vi "3-lorentzian-heat-response -- V4.vi"(7 "action":T2, 10 "Map IN":map{T1, dbl}(c390), 11 "omega IN (rad/sec)":dbl=0.1 format="%#_10f") -> (1 "Romega":cdb=0.1+0.0i format="%#_10f", 2 "Map OUT":map{T1, dbl}(c390), 3 "omega OUT(rad/sec)":dbl=0.1 format="%#_10f")   [LabVIEW 2020]
uses:
  3-lorentzian-heat-response action.ctl
  3-lorentzian-parameters.ctl
  142dd4c5-f9ed-c64b-bc14-a88e3e2c450a.vi
  <vilib>/Analysis/polynomials.llb/Polynomial Roots (DBL).vi
  <vilib>/Comparison/Less/Less Functor/Less Functor.lvclass
  <vilib>/Analysis/NI_AALPro.lvlib
panel:
  out "m1":dbl=0.1 format="%#_10f"
  out "m2":dbl=0.1 format="%#_10f"
  out "m3":dbl=0.1 format="%#_10f"
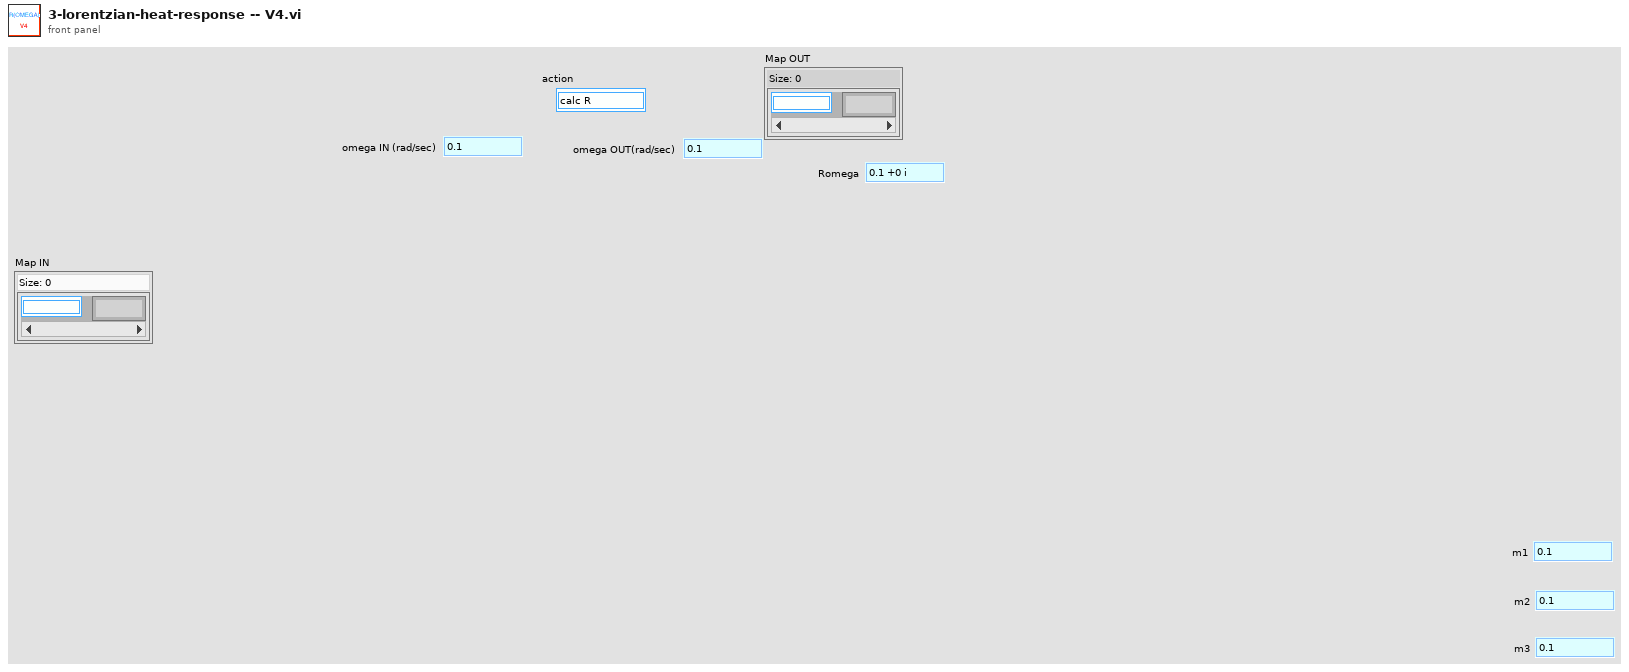
[diagram p1: front panel]
types:
  T1 = typedef "3-lorentzian-parameters.ctl" = enum16{"ζ", "τ1", "τS", "τN", "τC", "κ0", "m1", "m2", "m3", "T (K)", "B (T)", "θ (deg)", "side (S|R)", "set of (B|T)", "Re(offset)", "Im(offset)"}
  T2 = typedef "3-lorentzian-heat-response action.ctl" = enum16{"calc R", "create string", "calc m1m2m3", "dζ", "dT1", "dτS", "dτN", "dτC", "d-all", "dκ0", "T(K)", "m1", "m2", "m3", "parse string", "θ (deg)", "B (T)", "onlygrads", "newton", "create emty string"}
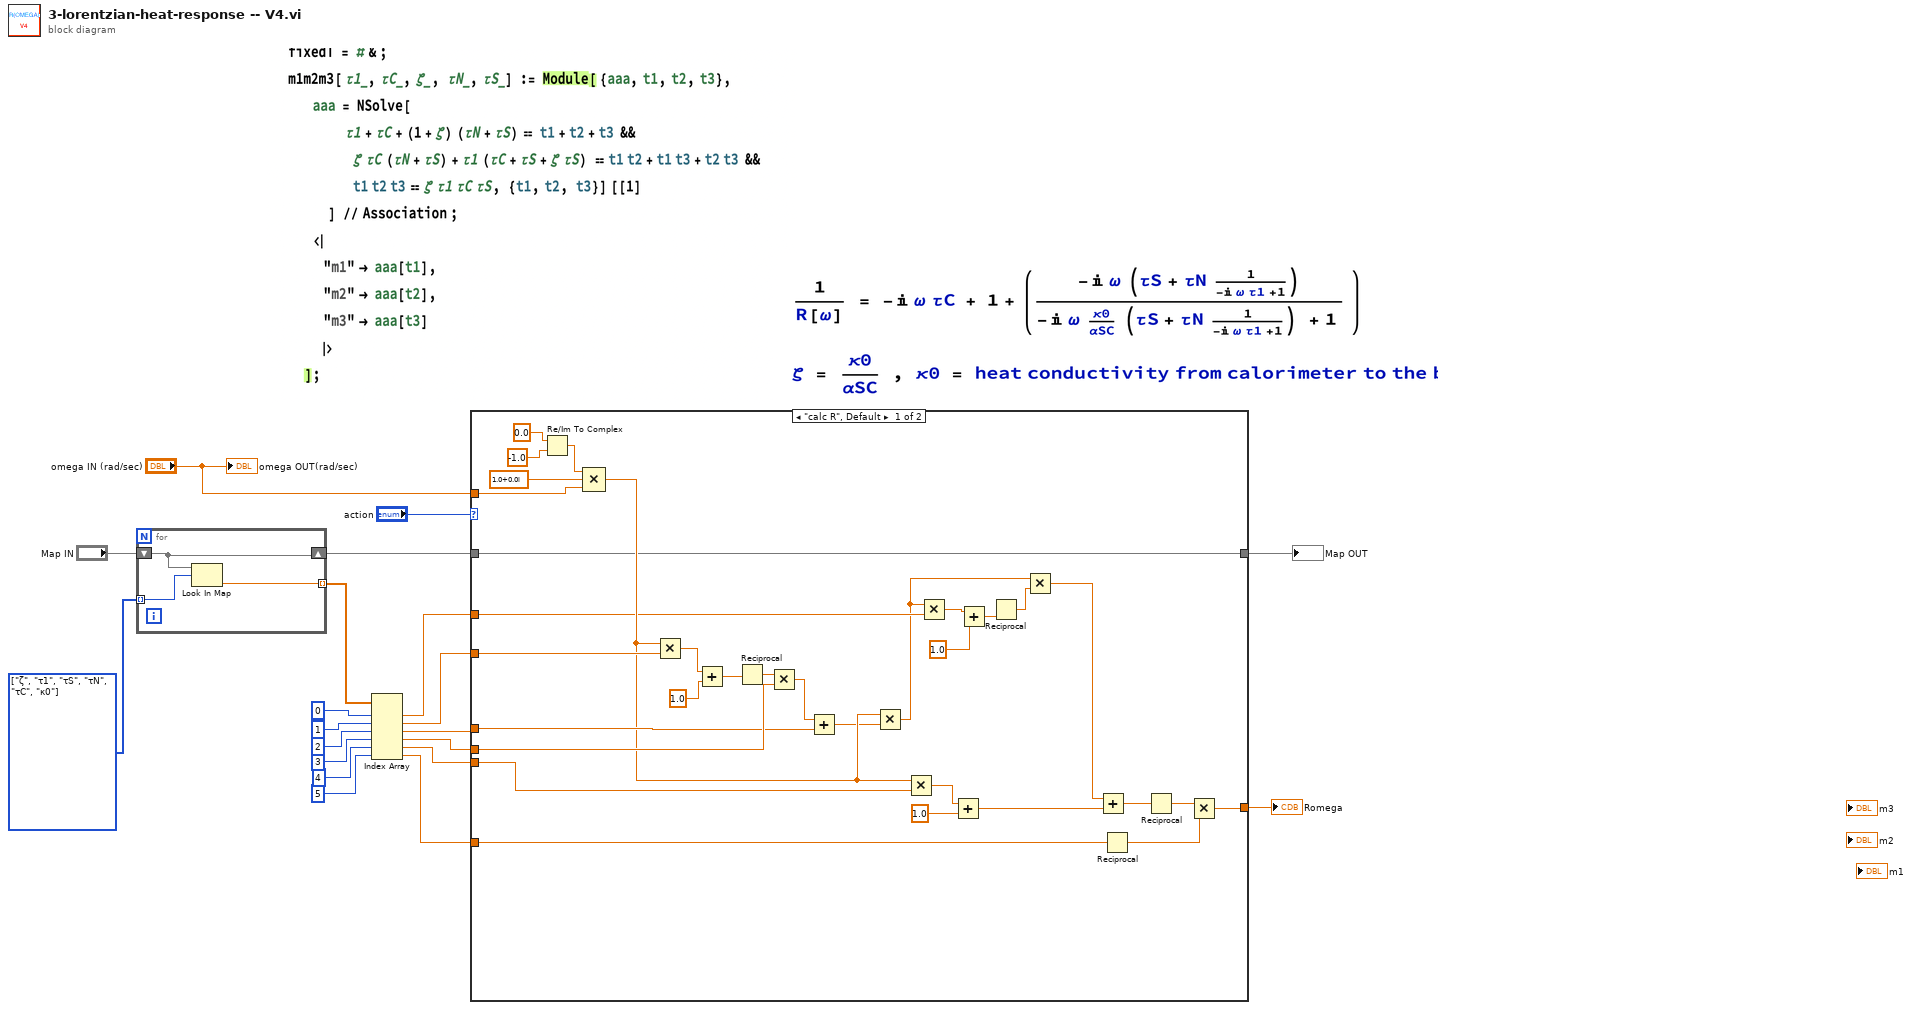
[diagram p0: block diagram]
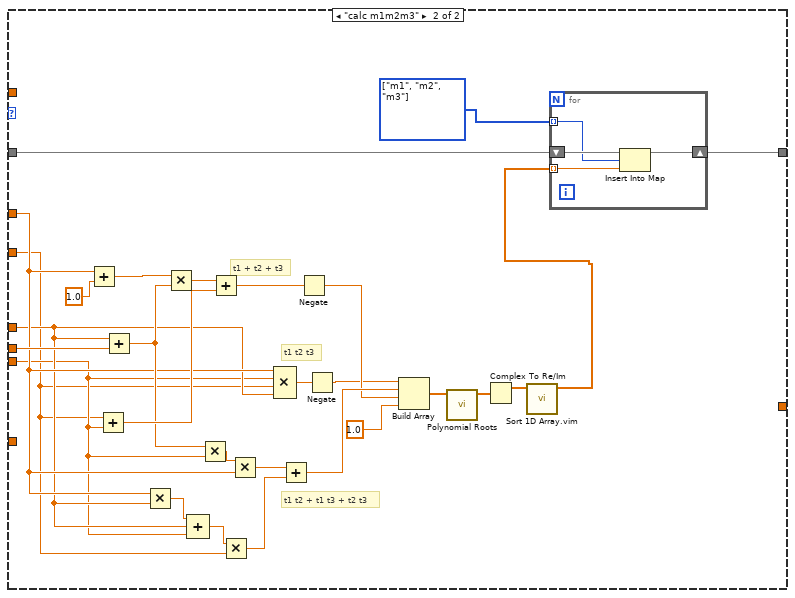
[diagram p2: hidden frame]
diagram:
  w5 = T1[] [enum."ζ", enum."τ1", enum."τS", enum."τN", enum."τC", enum."κ0"] items=["ζ", "τ1", "τS", "τN", "τC", "κ0", "m1", "m2", "m3", "T (K)", "B (T)", "θ (deg)", "side (S|R)", "set of (B|T)", "Re(offset)", "Im(offset)"]
  n1 = for {
    tunnel: w5 -> [w23] mode=indexing
    tunnel: [w22] -> w3 mode=indexing
    shift-right: [w21] -> w2
    shift-left: "Map IN" -> [w21]
    n2 = Look In Map(map=w21, key=w23) -> (value=w22:dbl)  [unwired: 1 in, 1 out]
  }
  n3 = Index Array(array=w3, index #1=0 ("index"), index #2=1 ("index"), index #3=2 ("index"), index #4=3 ("index"), index #5=4 ("index"), index #6=5 ("index")) -> (element #1=w12:dbl, element #2=w11:dbl, element #3=w10:dbl, element #4=w9:dbl, element #5=w8:dbl, element #6=w7:dbl)
  n4 = case shown="\"calc R\", Default" "action" {
    tunnel: w8 -> [w41 w69]
    tunnel: "omega IN (rad/sec)" -> [w44 _]
    tunnel: w11 -> [w43 w67]
    tunnel: w9 -> [w49 w82]
    tunnel: w10 -> [w47 w70]
    tunnel: w12 -> [w37 w72]
    tunnel: [w25 _] -> w19
    tunnel: w7 -> [w28 _]
    tunnel: [w24 w58] -> w1
    tunnel: w2 -> [w24 w59]
    frame "calc R", Default {
      n5 = Re/Im To Complex(1:-1.0 ("y"), 2:0.0 ("x")) -> (0:w45:cdb)
      n6 = Compound Arithmetic op=MULTIPLY(w45, cdb 1.0+0.0i ("value"), w44) -> (w39:cdb)
      n7 = Multiply(x=w39, y=w43) -> (x*y=w42:cdb)
      n8 = Add(x=w42, y=1.0) -> (x+y=w51:cdb)
      n9 = Reciprocal(x=w51) -> (1/x=w50:cdb)
      n10 = Multiply(x=w50, y=w49) -> (x*y=w48:cdb)
      n11 = Add(x=w48, y=w47) -> (x+y=w38:cdb)
      n12 = Multiply(x=w39, y=w38) -> (x*y=w33:cdb)
      n13 = Multiply(x=w39, y=w41) -> (x*y=w40:cdb)
      n14 = Multiply(x=w33, y=w37) -> (x*y=w35:cdb)
      n15 = Add(x=w40, y=1.0) -> (x+y=w31:cdb)
      n16 = Add(x=w35, y=1.0) -> (x+y=w34:cdb)
      n17 = Reciprocal(x=w34) -> (1/x=w32:cdb)
      n18 = Multiply(x=w33, y=w32) -> (x*y=w30:cdb)
      n19 = Add(x=w30, y=w31) -> (x+y=w29:cdb)
      n20 = Reciprocal(x=w28) -> (1/x=w26:dbl)
      n21 = Reciprocal(x=w29) -> (1/x=w27:cdb)
      n22 = Multiply(x=w27, y=w26) -> (x*y=w25:cdb)
    }
    frame "calc m1m2m3" {
      w57 = T1[] [enum."m1", enum."m2", enum."m3"] items=["ζ", "τ1", "τS", "τN", "τC", "κ0", "m1", "m2", "m3", "T (K)", "B (T)", "θ (deg)", "side (S|R)", "set of (B|T)", "Re(offset)", "Im(offset)"]
      # "t1 t2 + t1 t3 + t2 t3"
      # "t1 + t2 + t3"
      # "t1 t2 t3"
      n23 = Add(x=w72, y=1.0) -> (x+y=w81:dbl)
      n24 = Add(x=w67, y=w69) -> (x+y=w79:dbl)
      n25 = Add(x=w70, y=w82) -> (x+y=w74:dbl)
      n26 = Multiply(x=w72, y=w70) -> (x*y=w71:dbl)
      n27 = Multiply(x=w81, y=w74) -> (x*y=w80:dbl)
      n28 = Compound Arithmetic op=ADD(w71, w70, w69) -> (w68:dbl)
      n29 = Multiply(x=w74, y=w69) -> (x*y=w73:dbl)
      n30 = Add(x=w80, y=w79) -> (x+y=w75:dbl)
      n31 = Multiply(x=w68, y=w67) -> (x*y=w65:dbl)
      n32 = Multiply(x=w73, y=w72) -> (x*y=w66:dbl)
      n33 = Compound Arithmetic op=MULTIPLY(w72, w69, w67, w70) -> (w78:dbl)
      n34 = Add(x=w66, y=w65) -> (x+y=w64:dbl)
      n35 = Negate(x=w75) -> (-x=w61:dbl)
      n36 = Negate(x=w78) -> (-x=w60:dbl)
      n37 = Build Array(w60, w64, w61, 1.0 ("element")) -> (w76:dbl[])
      n38 = call-poly <vilib>:"Polynomial Roots.vi"("P(x)"=w76) -> ("Roots"=w63:cdb[])  [unwired: 9 in, 1 out]
      n39 = Complex To Re/Im(x + iy=w63) -> (x=w62:dbl[])  [unwired: 1 out]
      n40 = call "Sort 1D Array.vim"("unsorted array"=w62) -> ("sorted array"=w56:dbl[])  [unwired: 10 in]
      n41 = for {
        shift-right: [w86] -> w58
        shift-left: w59 -> [w87]
        tunnel: w57 -> [w85] mode=indexing
        tunnel: w56 -> [w84] mode=indexing
        n42 = Insert Into Map(map in=w87, key=w85, value=w84) -> (map out=w86:map{T1, dbl})  [unwired: 2 out]
      }
    }
  }
  "Romega" <- w19
  "Map OUT" <- w1
  "omega OUT(rad/sec)" <- "omega IN (rad/sec)"
